vi "Apply Item Symbols.vi"(8 "error in (no error)":errorcluster, 11 "Selector in":refnum<class "Selector.lvclass">) -> (0 "error out":errorcluster, 3 "Selector out":refnum<class "Selector.lvclass">)   [LabVIEW 2019, in "Selector.lvclass"]
uses:
  Selector.lvclass
  Selector.lvclass/Selector.ctl
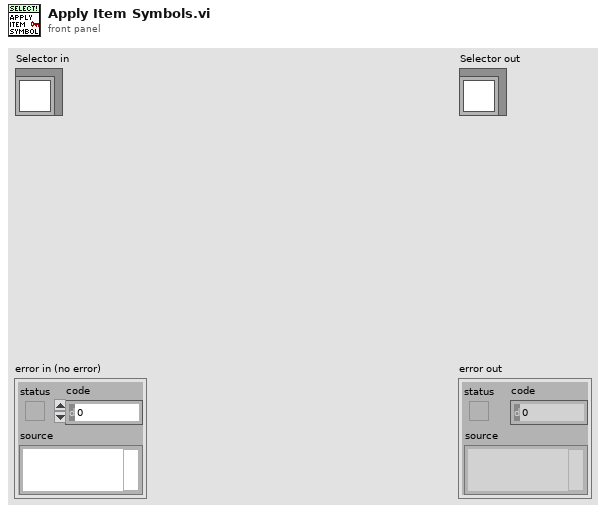
[diagram p1: front panel]
types:
  T1 = typedef "Selector.lvclass/Item.ctl" = cluster{"Name":string, "Group":string, "Enabled":bool}
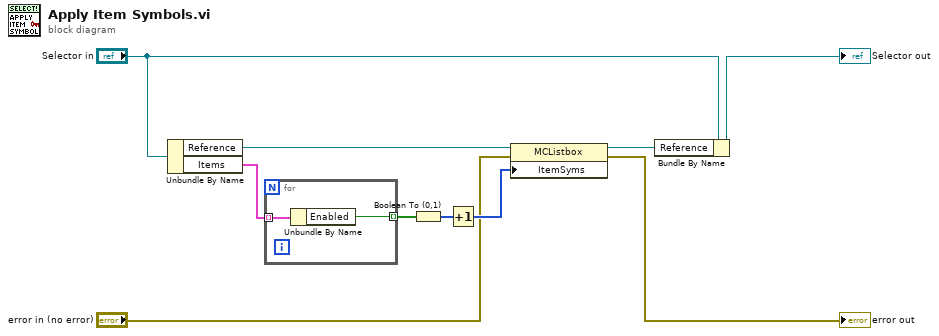
[diagram p0: block diagram]
diagram:
  n1 = Unbundle By Name("Selector in") -> ("Reference"=w10:refnum<vi>, "Items"=w2:T1[])
  n2 = for {
    tunnel: w2 -> [w12] mode=indexing
    tunnel: [w11] -> w1 mode=indexing
    n3 = Unbundle By Name(w12) -> ("Enabled"=w11:bool)
  }
  n4 = Boolean To (0,1)(Boolean=w1) -> (0, 1=w9:i16[])
  n5 = Increment(x=w9) -> (x+1=w8:i16[])
  n6 = property class="MCListbox"(reference=w10, error in="error in (no error)", "ItemSyms"=w8) -> (reference out=w5:refnum<vi>, error out=→"error out":errorcluster)
  n7 = Bundle By Name(cluster="Selector in", "Reference"=w5) -> (→"Selector out":refnum<class "Selector.lvclass">)
